vi "Transform Cluster Update.vi"(4 "Axis":enum16{"X-Scale", "Y-Scale", "Z-Scale"}(ring), 6 "NewRange":T6, 7 "Multiplot Representation In":T1, 8 "error in (no error)":errorcluster, 10 "Actual Transform In":T5, 11 "3D Plot in":refnum<class "3D Plot.lvclass">) -> (0 "error out":errorcluster, 2 "Actual Transform Out":T5, 3 "3D Plot out":refnum<class "3D Plot.lvclass">, 5 "Multiplot Representation Out":T1)   [LabVIEW 2017, in "3D Plot.lvclass"]
uses:
  <vilib>/Math Plots/3D Math Plots/3D Plot/3D Plot/3D Plot.lvclass
  <vilib>/Math Plots/3D Math Plots/3D Plot/3D Plot/Typedef/Actual Transform.ctl
  <vilib>/Math Plots/3D Math Plots/3D Plot/3D Plot/Typedef/Range Clusters.ctl
  <vilib>/Math Plots/3D Math Plots/3D Plot/3D Plot/Typedef/Multiplot Representation.ctl
  <vilib>/Math Plots/3D Math Plots/3D Plot/3D Plot/Typedef/Plot Representation.ctl
  <vilib>/Math Plots/3D Math Plots/3D Plot/3D Plot/Typedef/Mesh Data.ctl
  <vilib>/Math Plots/3D Math Plots/3D Plot/3D Plot/3D Plot.lvclass/3D Plot.ctl
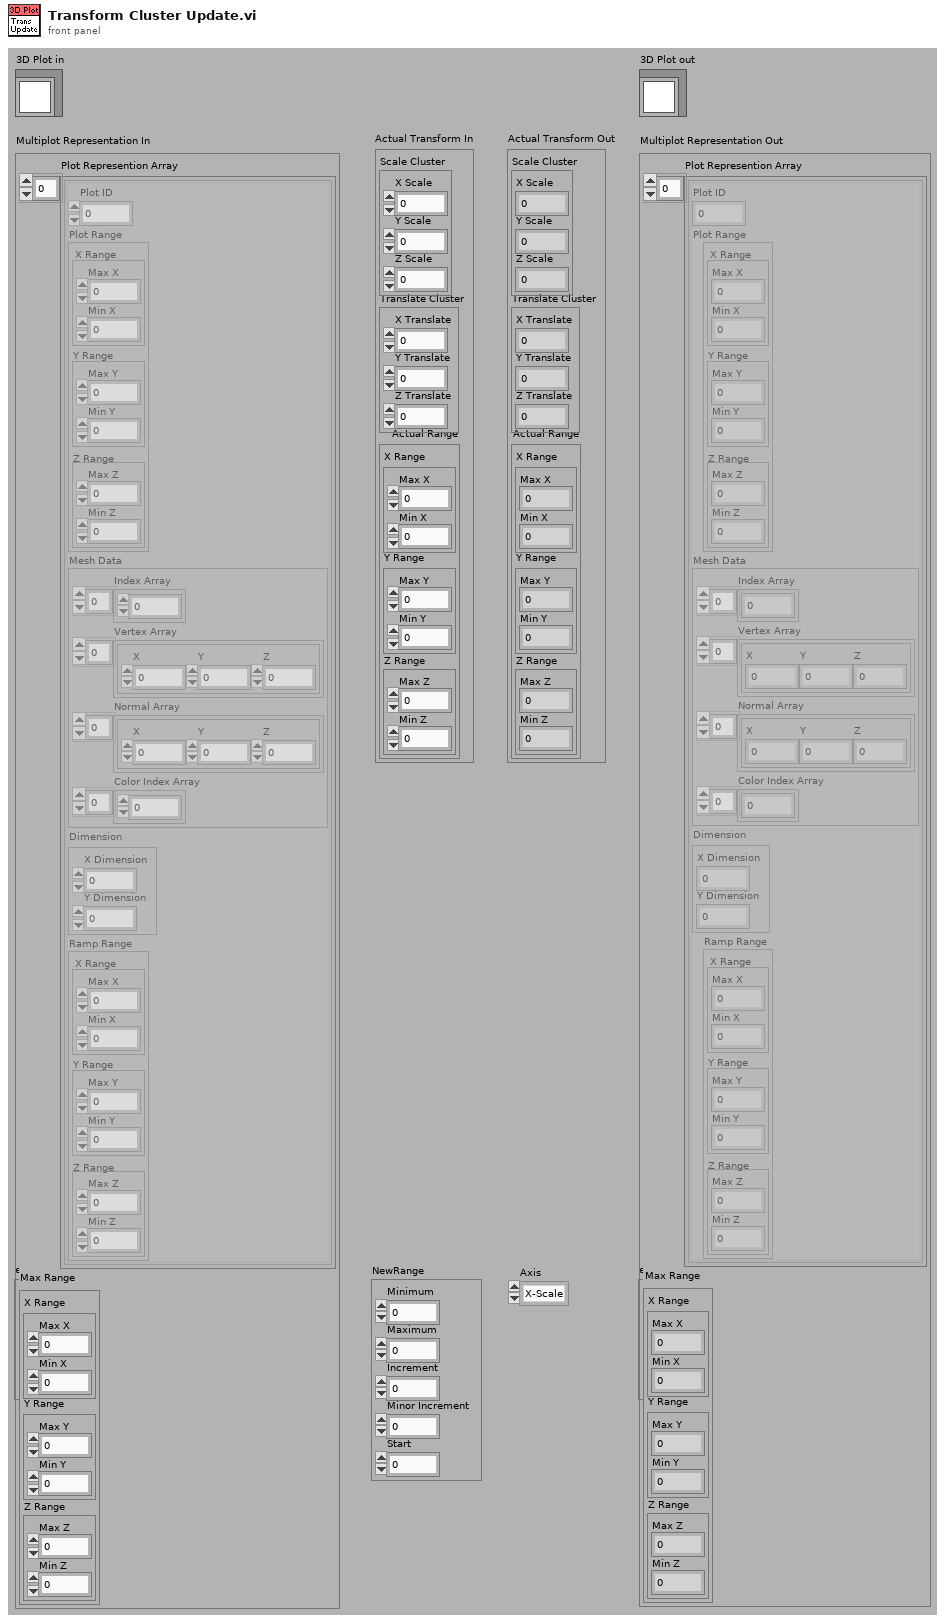
[diagram p1: front panel]
types:
  T1 = typedef "3D Plot.lvclass/Multiplot Representation.ctl" = cluster{"Plot Represention Array":T2[], "Max Range":T3}
  T2 = typedef "3D Plot.lvclass/Plot Representation.ctl" = cluster{"Plot ID":i32, "Plot Range":T3, "Mesh Data":T4, "Dimension":cluster{"X Dimension":i32, "Y Dimension":i32}, "Ramp Range":T3}
  T3 = typedef "3D Plot.lvclass/Range Clusters.ctl" = cluster{"X Range":cluster{"Max X":sgl, "Min X":sgl}, "Y Range":cluster{"Max Y":sgl, "Min Y":sgl}, "Z Range":cluster{"Max Z":sgl, "Min Z":sgl}}
  T4 = typedef "3D Plot.lvclass/Mesh Data.ctl" = cluster{"Index Array":u32[], "Vertex Array":cluster{"X":sgl, "Y":sgl, "Z":sgl}[], "Normal Array":cluster{"X":sgl, "Y":sgl, "Z":sgl}[], "Color Index Array":i32[]}
  T5 = typedef "3D Plot.lvclass/Actual Transform.ctl" = cluster{"Scale Cluster":cluster{"X Scale":sgl, "Y Scale":sgl, "Z Scale":sgl}, "Translate Cluster":cluster{"X Translate":sgl, "Y Translate":sgl, "Z Translate":sgl}, "Actual Range":T3}
  T6 = cluster{"Minimum":dbl, "Maximum":dbl, "Increment":dbl, "Minor Increment":dbl, "Start":dbl}
  T7 = typedef "3D Plot.lvclass/Range Property.ctl" = cluster{"Range Cluster":T3, "Auto Range":cluster{"Auto Range X":bool, "Auto Range Y":bool, "Auto Range Z":bool}, "Inverted":cluster{"Inverted X":bool, "Inverted Y":bool, "Inverted Z":bool}, "Logarithm":cluster{"Logarithm X":bool, "Logarithm Y":bool, "Logarithm Z":bool}}
  T8 = cluster{"Logarithm X":bool, "Logarithm Y":bool, "Logarithm Z":bool}
  T9 = cluster{"Range Out":cluster{"Max":sgl, "Min":sgl}, "Range Out":cluster{"Max":sgl, "Min":sgl}, "Range Out":cluster{"Max":sgl, "Min":sgl}}
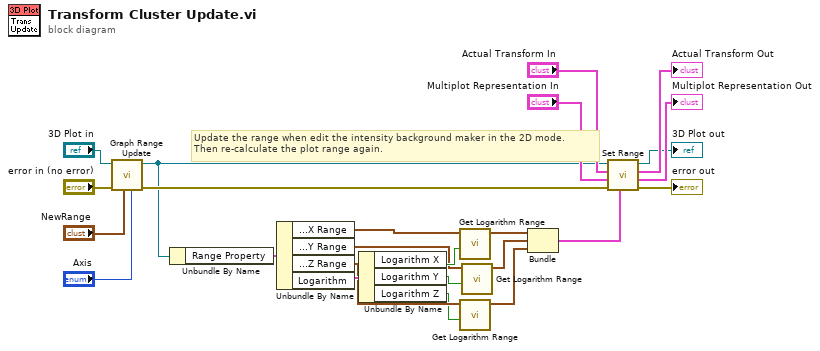
[diagram p0: block diagram]
diagram:
  # "Update the range when edit the intensity background maker in the 2D mode.\nThen re-calculate the plot range again."
  n1 = call <vilib>:"Graph Range Update.vi"("Axis"="Axis", "NewRange"="NewRange", "error in (no error)"="error in (no error)", "3D Plot.lvclass in"="3D Plot in") -> ("error out"=w17:errorcluster, "3D Plot.lvclass out"=w5:refnum<class "3D Plot.lvclass">)  [unwired: 2 in, 4 out]
  n2 = Unbundle By Name(w5) -> ("Range Property"=w13:T7)
  n3 = Unbundle By Name(w13) -> ("Range Cluster.X Range"=w12:cluster{"Max X":sgl, "Min X":sgl}, "Range Cluster.Y Range"=w10:cluster{"Max Y":sgl, "Min Y":sgl}, "Range Cluster.Z Range"=w9:cluster{"Max Z":sgl, "Min Z":sgl}, "Logarithm"=w15:T8)
  n4 = Unbundle By Name(w15) -> ("Logarithm X"=w11:bool, "Logarithm Y"=w7:bool, "Logarithm Z"=w8:bool)
  n5 = call <vilib>:"Get Logarithm Range.vi"("Logarithm?"=w11, "Range In"=w12) -> ("Range Out"=w4:cluster{"Max":sgl, "Min":sgl})  [unwired: 3 in, 6 out]
  n6 = call <vilib>:"Get Logarithm Range.vi"("Logarithm?"=w8, "Range In"=w9) -> ("Range Out"=w2:cluster{"Max":sgl, "Min":sgl})  [unwired: 3 in, 6 out]
  n7 = call <vilib>:"Get Logarithm Range.vi"("Logarithm?"=w7, "Range In"=w10) -> ("Range Out"=w3:cluster{"Max":sgl, "Min":sgl})  [unwired: 3 in, 6 out]
  n8 = Bundle("Range Out"=w4, "Range Out"=w3, "Range Out"=w2) -> (w1:T9)  [unwired: 1 out]
  n9 = call <vilib>:"Set Range.vi"("Range Cluster"=w1, "error in (no error)"=w17, "Multiplot Representation In"="Multiplot Representation In", "Actual Transform In"="Actual Transform In", "3D Plot.lvclass in"=w5) -> ("error out"=→"error out":errorcluster, "Multiplot Representation In"=→"Multiplot Representation Out":T1, "Actual Transform Out"=→"Actual Transform Out":T5, "3D Plot.lvclass out"=→"3D Plot out":refnum<class "3D Plot.lvclass">)  [unwired: 3 out]
